vi "Untitled 1 (SubVI).vi"(10 "Boolean 3":bool, 11 "Boolean in":bool) -> (3 "Boolean out":bool)   [LabVIEW 2021]
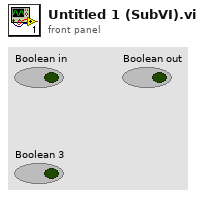
[diagram p1: front panel]
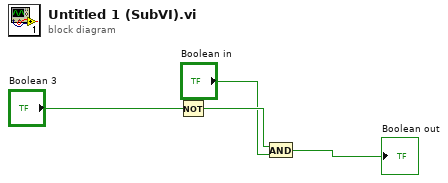
[diagram p0: block diagram]
diagram:
  n1 = Not(x="Boolean 3") -> (.not. x?=w3:bool)
  n2 = And(x=w3, y="Boolean in") -> (x .and. y?=→"Boolean out":bool)
